vi "Restart LV Dialog.vi"() -> ()   [LabVIEW 2011]
uses:
  USER32.DLL
panel:
  in  "Ok":bool
  # "You must restart LabVIEW after completing this installation to enable LINX features."
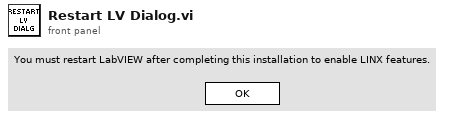
[diagram p1: front panel]
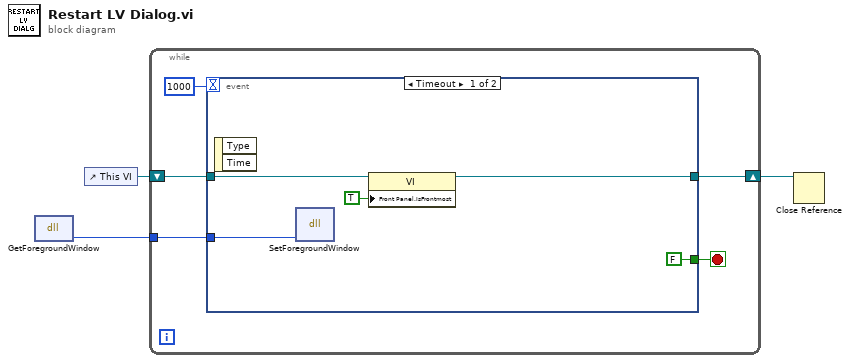
[diagram p0: block diagram]
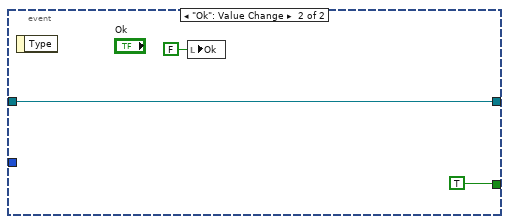
[diagram p2: hidden frame]
diagram:
  n1 = dll-call lib="USER32.DLL" fn="GetForegroundWindow"() -> ("return type"=w1:i32)  [unwired: 3 in, 2 out]
  n2 = control-ref of="This VI"() -> (w2:refnum<vi>)
  n3 = while {
    shift-right: [w6] -> w3
    shift-left: w2 -> [w5]
    tunnel: w1 -> [w4]
    stop <- w7 stop-if-true
    n4 = event shown="[0] Timeout" {
      selector: _ -> [_ _]
      dyn-events: _ -> [_ _]
      timeout: 1000 -> [_ _]
      tunnel: [FALSE ("Ok") TRUE ("Ok")] -> w7
      tunnel: [w10 w14] -> w6
      tunnel: w5 -> [w11 w14]
      tunnel: w4 -> [w9 _]
      event Timeout {
        n5 = event-data() -> ()  [unwired: 1 in, 2 out]
        n6 = dll-call lib="USER32.DLL" fn="SetForegroundWindow"("hwnd"=w9) -> ()  [unwired: 4 in, 3 out]
        n7 = property class="VI"(reference=w11, "Front Panel.IsFrontmost"=TRUE ("Front Panel Window:Is Frontmost")) -> (reference out=w10:refnum<vi>)  [unwired: 1 in, 1 out]
      }
      event "Ok": Value Change {
        n8 = event-data() -> ()  [unwired: 1 in, 1 out]
        n9 = local write "Ok"(FALSE ("Ok")) -> ()
      }
    }
  }
  n10 = Close Reference(reference=w3) -> ()  [unwired: 1 in, 1 out]
